vi "Print Buffer.vi"(5 "End Index (1)":u32=1, 6 "Byte Count (1024)":u32=2048, 7 "Start Index (1)":u32=1, 8 "error in (no error)":errorcluster, 9 "Buffer Name(s)":string, 11 "VISA resource name":refnum<visa-resource-name>) -> (0 "error out":errorcluster, 1 "Command String":string, 2 "Buffer Data":string, 3 "VISA resource name out":refnum<visa-resource-name>, 4 "Return Count":u32)   [LabVIEW 2018, in "Keithley 3706.lvlib"]
uses:
  <instrlib>/Keithley 3706/Keithley 3706.lvlib
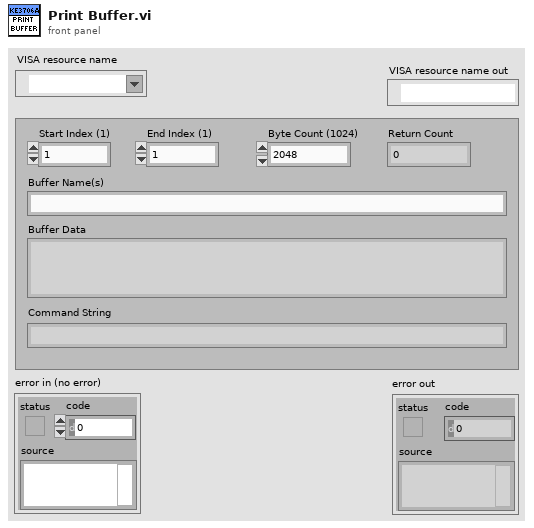
[diagram p1: front panel]
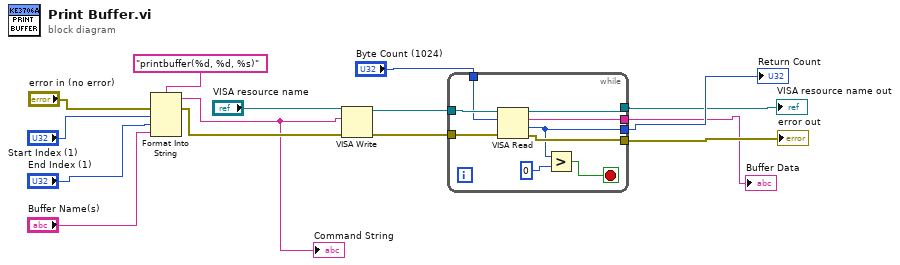
[diagram p0: block diagram]
diagram:
  n1 = Format Into String(format string="printbuffer(%d, %d, %s)", error in="error in (no error)", "Start Index (1)", "End Index (1)", "Buffer Name(s)") -> (resulting string=w8:string, error out=w9:errorcluster)  [unwired: 1 in]
  "Command String" <- w8
  n2 = VISA Write(VISA resource name="VISA resource name", write buffer=w8, error in (no error)=w9) -> (VISA resource name out=w7:refnum<visa-resource-name>, error out=w6:errorcluster)  [unwired: 1 out]
  n3 = while {
    tunnel: w7 -> [w24]
    tunnel: w6 -> [w23]
    tunnel: "Byte Count (1024)" -> [w22]
    tunnel: [w21] -> w2
    tunnel: [w20] -> w1
    tunnel: [w18] -> w3
    tunnel: [w19] -> w4
    stop <- w16 stop-if-true
    n4 = VISA Read(VISA resource name=w24, byte count=w22, error in (no error)=w23) -> (VISA resource name out=w21:refnum<visa-resource-name>, read buffer=w20:string, return count=w18:u32, error out=w19:errorcluster)
    n5 = Greater?(x=w18, y=0) -> (0:w16:bool)
  }
  "VISA resource name out" <- w2
  "error out" <- w4
  "Buffer Data" <- w1
  "Return Count" <- w3
